vi "ini_zeros.vi"() -> (1 "Array 4":dbl[](array[numeric]), 2 "Array 3":dbl[](array[numeric]), 3 "Array 2":dbl[][](array[numeric]), 4 "Array":dbl[](array[numeric]))   [LabVIEW 2013]
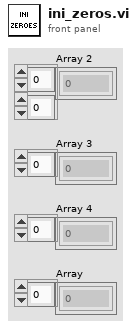
[diagram p1: front panel]
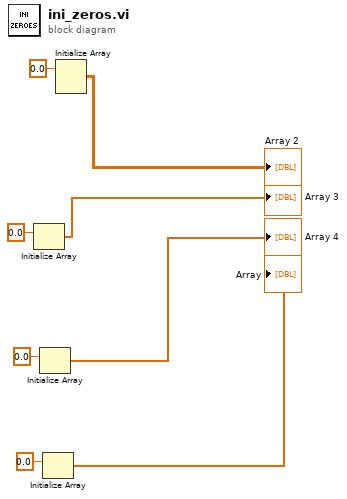
[diagram p0: block diagram]
diagram:
  n1 = Initialize Array(0.0 ("element")) -> (→"Array 3":dbl[])  [unwired: 1 in]
  n2 = Initialize Array(0.0 ("element")) -> (→"Array 4":dbl[])  [unwired: 1 in]
  n3 = Initialize Array(0.0 ("element")) -> (→"Array":dbl[])  [unwired: 1 in]
  n4 = Initialize Array(0.0 ("element")) -> (→"Array 2":dbl[][])  [unwired: 2 in]
